vi "Get Channel Names and Default Values.vi"(8 "error in":errorcluster, 10 "channels":refnum<class "Channel.lvclass">[](array[class]), 11 "counter driven output mode in":refnum<class "Counter Driven Output Mode.lvclass">) -> (0 "error out":errorcluster, 1 "default values":dbl[](array[numeric]), 2 "names":string[](array[string]), 3 "counter driven output mode out":refnum<class "Counter Driven Output Mode.lvclass">)   [LabVIEW 2017, in "Scan Engine Scripting.lvlib" / "Counter Driven Output Mode.lvclass"]
uses:
  Counter Driven Output Mode.lvclass
  Channel Classes/Channel/Channel.lvclass
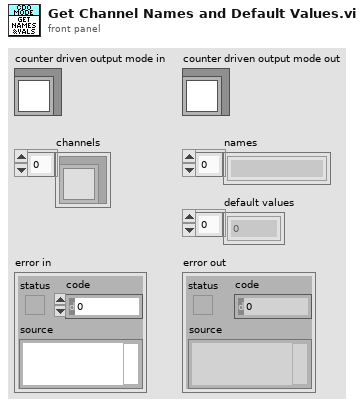
[diagram p1: front panel]
types:
  T1 = typedef "Scan Engine Scripting.lvlib/counter driven output channel settings.ctl" = cluster{"name":string, "default value":bool, "counter driven state":T2}
  T2 = typedef "Scan Engine Scripting.lvlib/Counter Driven Output Channel.lvclass/Counter Driven State.ctl" = enum16{"Disabled", "Enabled"}
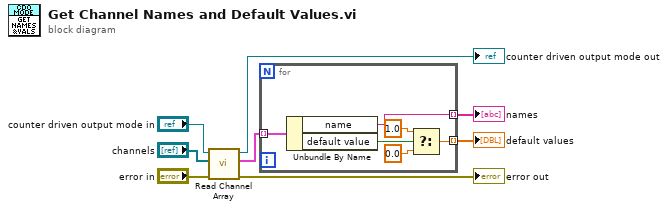
[diagram p0: block diagram]
diagram:
  n1 = call "Read Channel Array.vi"("error in"="error in", "channels"="channels", "counter driven output mode in"="counter driven output mode in") -> ("error out"=→"error out":errorcluster, "channel settings"=w5:T1[], "counter driven output mode out"=→"counter driven output mode out":refnum<class "Counter Driven Output Mode.lvclass">)  [unwired: 6 in]
  n2 = for {
    tunnel: w5 -> [w14] mode=indexing
    tunnel: [w10] -> w2 mode=indexing
    tunnel: [w9] -> w3 mode=indexing
    n3 = Unbundle By Name(w14) -> ("name"=w10:string, "default value"=w12:bool)
    n4 = Select(t=1.0, s=w12, f=0.0) -> (s? t:f=w9:dbl)
  }
  "names" <- w2
  "default values" <- w3
